vi "Read configuration item.vi"(8 "error in (no error)":errorcluster, 10 "configuration item":string, 11 "IConfigDBQueries in":refnum<class "sqlite-queries.lvclass">) -> (0 "error out":errorcluster, 2 "resulting string":string)   [LabVIEW 2020, in "sqlite-queries.lvlib" / "sqlite-queries.lvclass"]
uses:
  sqlite-queries.lvclass
  sqlite-queries.lvclass/sqlite-queries.ctl
  externals/database-interface/IDatabase/IDatabase.lvlib
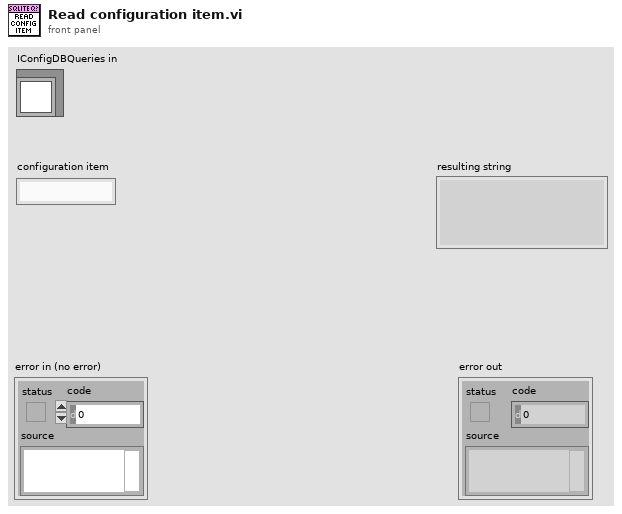
[diagram p1: front panel]
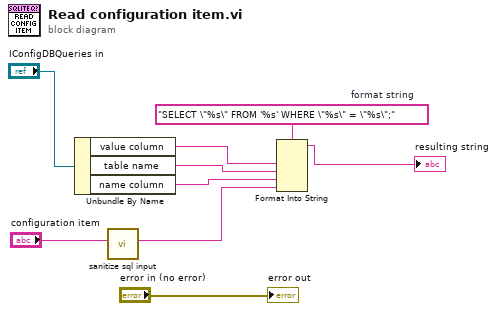
[diagram p0: block diagram]
diagram:
  w8 = "SELECT \"%s\" FROM '%s' WHERE \"%s\" = \"%s\";"  # format string
  n1 = Unbundle By Name("IConfigDBQueries in") -> ("value column"=w2:string, "table name"=w3:string, "name column"=w4:string)
  n2 = call "sanitize sql input.vi"("Sting in"="configuration item") -> ("String out"=w1:string)  [unwired: 8 in, 2 out]
  n3 = Format Into String(format string=w8, w2, w3, w4, w1) -> (resulting string=→"resulting string":string)  [unwired: 2 in, 1 out]
  "error out" <- "error in (no error)"
